vi "svx_Timebase Attribute.vi"(11 "attribute":variant) -> (0 "order":string, 1 "pair":string, 2 "samples/rev":dbl)   [LabVIEW 2017, in "SVX Timebase.xctl"]
uses:
  <vilib>/addons/_XControls/Timebase Plot/SVX Timebase.xctl
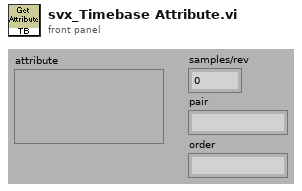
[diagram p1: front panel]
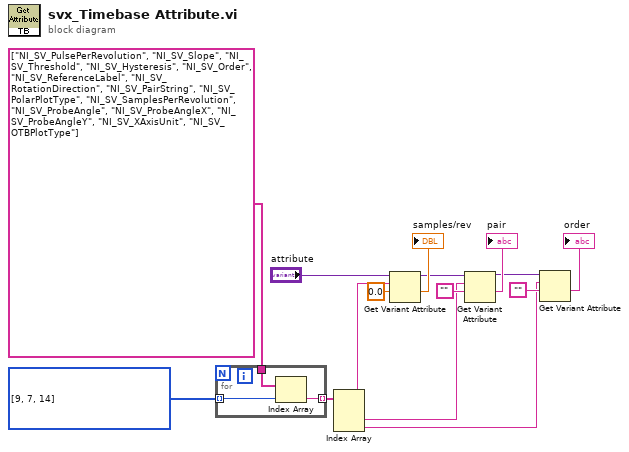
[diagram p0: block diagram]
diagram:
  w5 = u16[] [9, 7, 14] items=["Pulse / Revolution", "Slope", "Threshold", "Hysteresis", "Order", "Reference Label", "Rotation Direction", "Pair String", "Polar Plot Type", "Sample Per Revolution", "Probe Angle", "Probe Angle X", "Probe Angle Y", "X Axis Unit", "OTB Plot Type"]
  n1 = for {
    tunnel: string[] ["NI_SV_PulsePerRevolution", "NI_SV_Slope", "NI_SV_Threshold", "NI_SV_Hysteresis", "NI_SV_Order", "NI_SV_ReferenceLabel", "NI_SV_RotationDirection", "NI_SV_PairString", "NI_SV_PolarPlotType", "NI_SV_SamplesPerRevolution", "NI_SV_ProbeAngle", "NI_SV_ProbeAngleX", "NI_SV_ProbeAngleY", "NI_SV_XAxisUnit", "NI_SV_OTBPlotType"] -> [w18]
    tunnel: w5 -> [w17] mode=indexing
    tunnel: [w16] -> w4 mode=indexing
    n2 = Index Array(array=w18, index=w17) -> (element=w16:string)
  }
  n3 = Index Array(array=w4) -> (element #1=w3:string, element #2=w2:string, element #3=w1:string)  [unwired: 3 in]
  n4 = Get Variant Attribute(Variant="attribute", name=w3, default value (empty Variant)=0.0 ("pair")) -> (duplicate Variant=w14:variant, value=→"samples/rev":dbl)  [unwired: 1 in, 2 out]
  n5 = Get Variant Attribute(Variant=w14, name=w2, default value (empty Variant)="") -> (duplicate Variant=w10:variant, value=→"pair":string)  [unwired: 1 in, 2 out]
  n6 = Get Variant Attribute(Variant=w10, name=w1, default value (empty Variant)="") -> (value=→"order":string)  [unwired: 1 in, 3 out]
